vi "GUI_TEA_HPD.vi"() -> ()   [LabVIEW 2013]
uses:
  shared programs/GUI_Template/GUI_master/tcp_new_data_event.ctl
  shared programs/GUI_Template/GUI_master/tcp new data cluster.ctl
  General/shared/Image GUI options.ctl
  Device Driver/FilterWheels/posTypDef.ctl
panel:
  in  "pos.Channel2::6":T1=enum."3" caption="M3_HPD near FilterWheel"
  in  "pos.Channel1::6":T1=enum."3" caption="M3_HPD FilterWheel"
  in  "GUIdevice 6":string="BELLA_filter_wheels"
  in  "Target.X::2":dbl=0.001 caption="X" min=0.0 max=2000.0
  in  "Target.Y::2":dbl=0.001 caption="Y" min=0.0 max=2000.0
  in  "size2":dbl=25.0 caption="Size" min=0.0 max=0.0
  in  "Target.X::5":dbl=0.001 caption="X" min=0.0 max=2000.0
  in  "Target.Y::5":dbl=0.001 caption="Y" min=0.0 max=2000.0
  in  "size5":dbl=25.0 caption="Size" min=0.0 max=0.0
  in  "Image options":T2
  in  "Image options":T2
  in  "GUIdevice 1":string="BELLA_TEA_PowerMeter"
  in  "Reading::1":dbl=0.5 caption="Power (W)" min=0.0 max=50000.0 format="%_4p"
  in  "stop":bool
  out "power":dbl=9999.0 caption="Power (W)" min=0.0 max=300000000.0 format="%_4p"
  in  "Clear":bool
  out "XY Graph":cluster{dbl[], dbl[]}(graph)
  in  "trigger::2":bool caption="Blank Button"
  in  "exposure::2":dbl=0.001 caption="Exposure" min=3.8e-05 max=1.0 format="%_4p"
  out "Display2":T3(plugin-control) caption="M3HPD_CCD"
  in  "GUIdevice 2":string="M3HPD_CCD"
  out "image::2":T3(plugin-control) caption="M1 Cam"
  in  "trigger::5":bool caption="Blank Button"
  in  "exposure::5":dbl=0.001 caption="Exposure" min=3.8e-05 max=1.0 format="%_4p"
  out "Display5":T3(plugin-control) caption="M3HPD_CCD_Near"
  in  "GUIdevice 5":string="M3HPD_CCD_Near"
  out "image::5":T3(plugin-control) caption="M1 Cam"
  out "error IO 2":errorcluster
  out "tcp data event":T4
  # "BELLA TEA HPD MAP"
  # "TEA Power Meter"
  # "Target"
  # "Target"
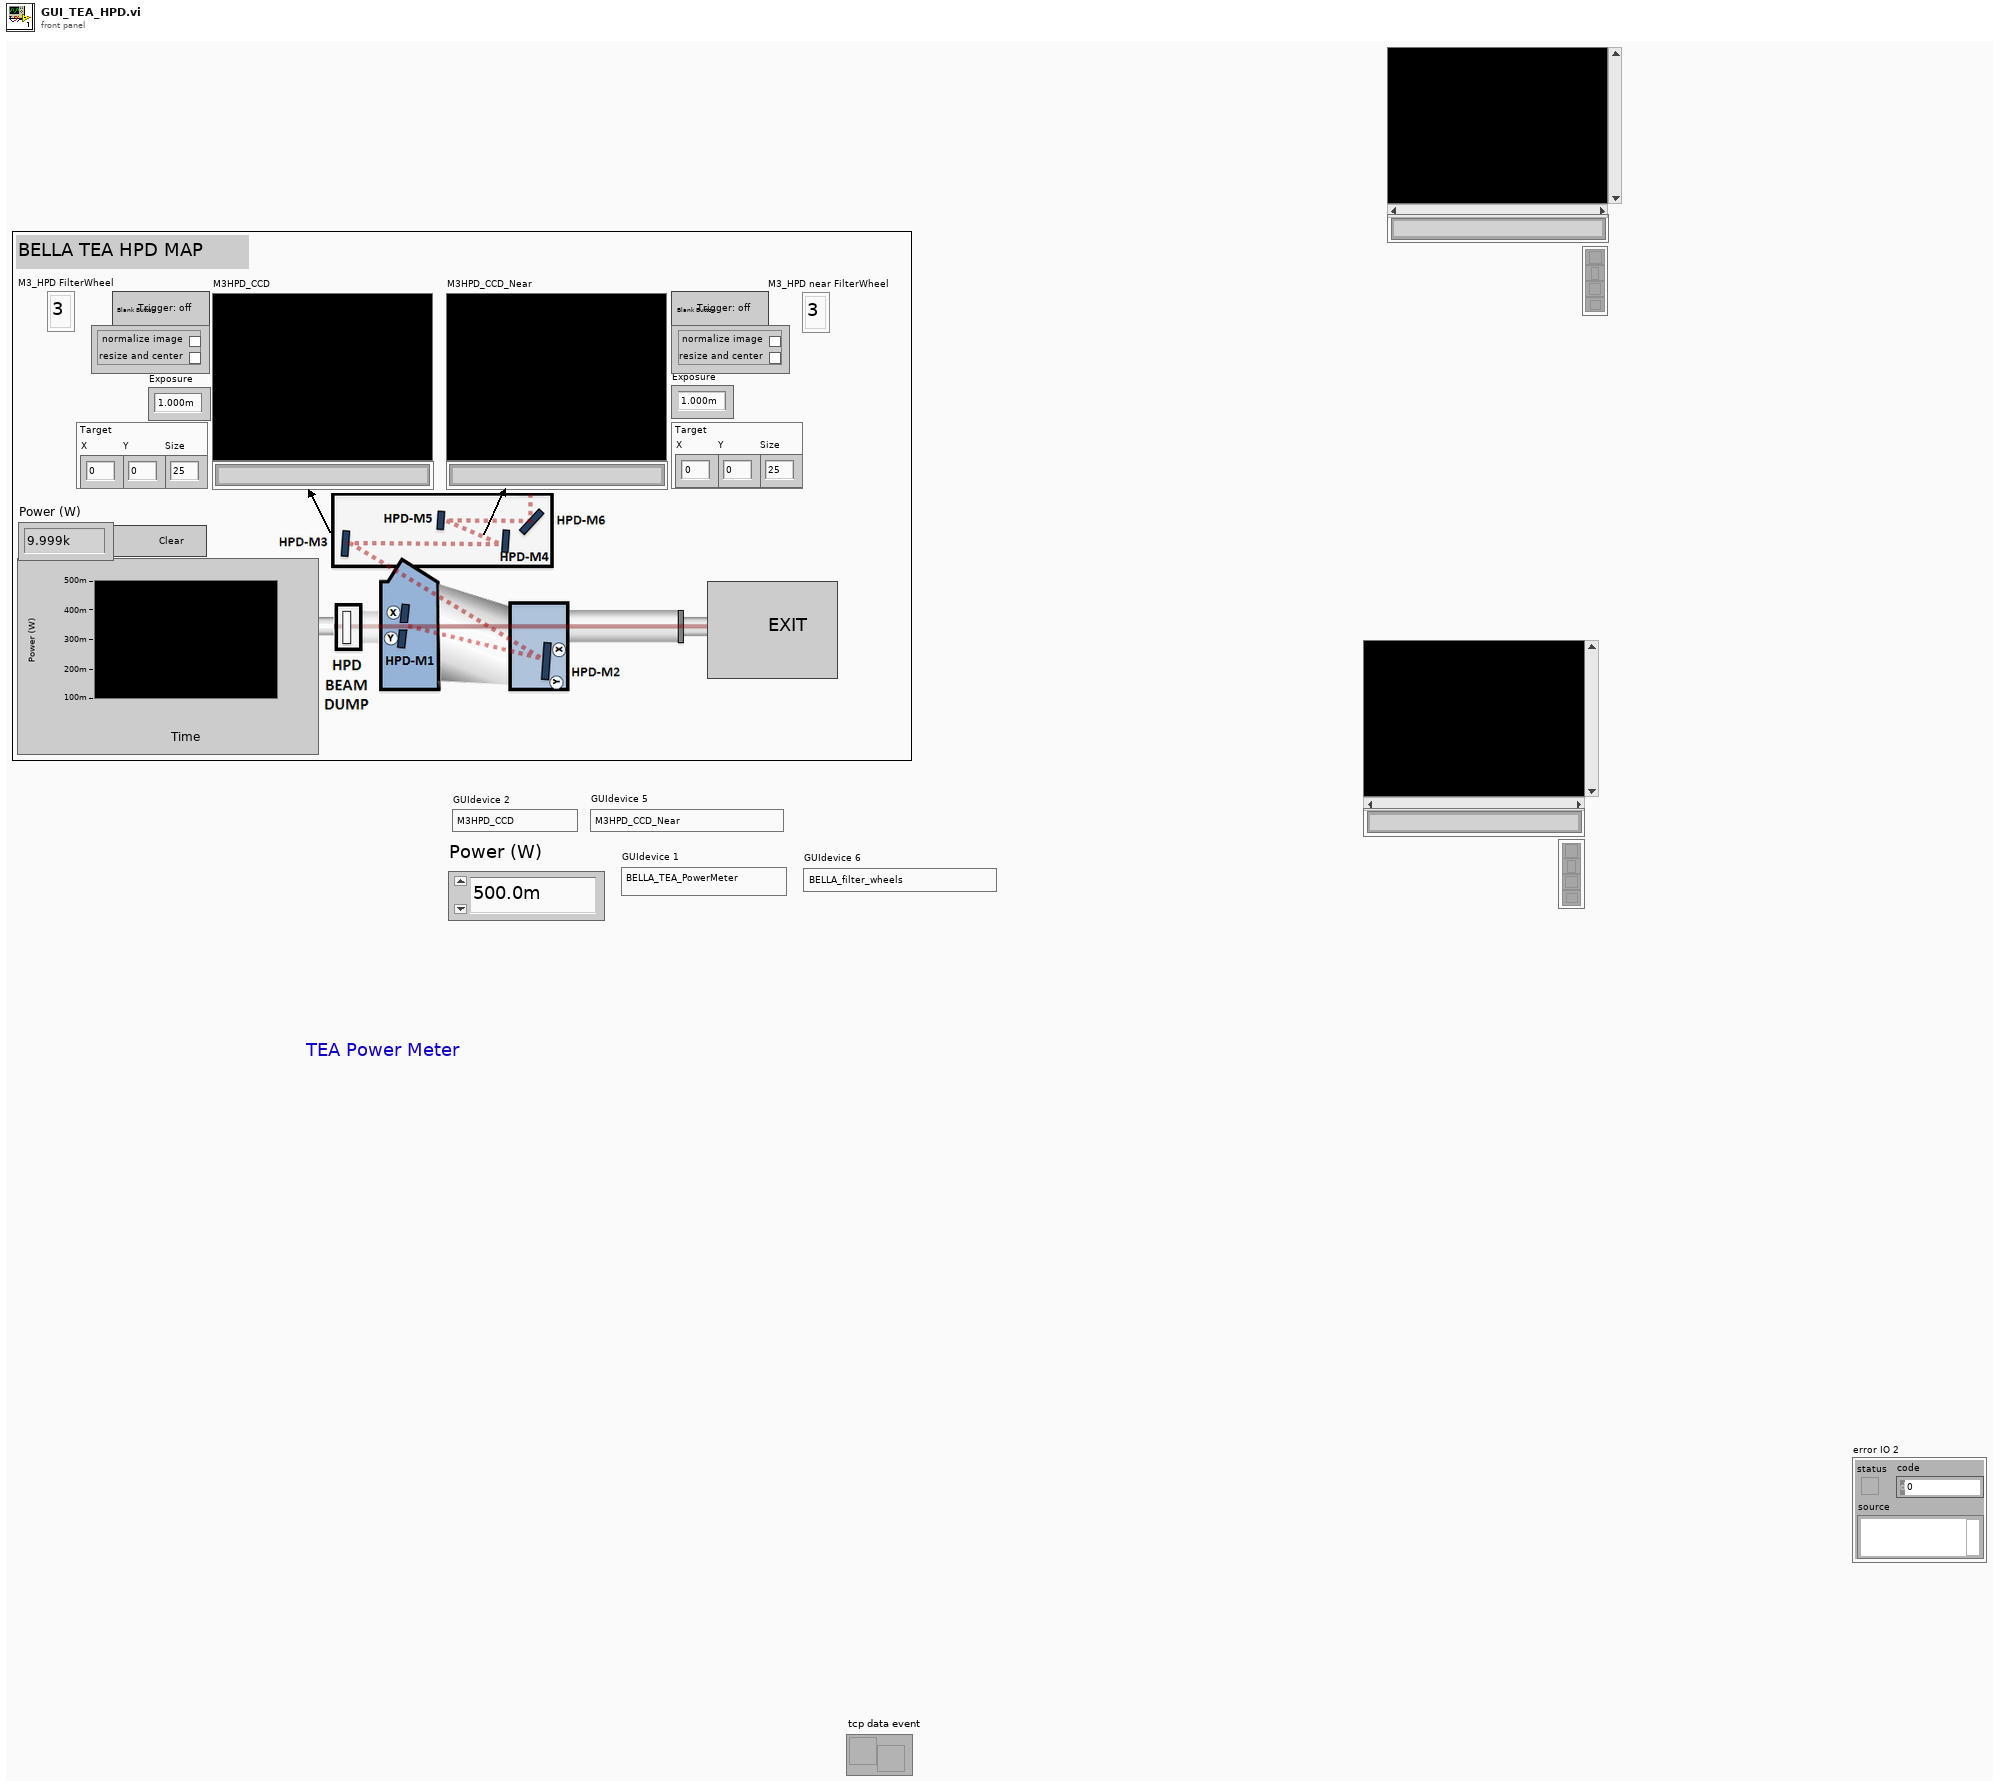
[diagram p1: front panel]
types:
  T1 = typedef "posTypDef.ctl" = enum16{"1", "2", "3", "4", "5", "6"}
  T2 = typedef "Image GUI options.ctl" = cluster{"normalize image":bool, "resize and center":bool}
  T3 = typedef "IMAQ Image.ctl" = refnum<image>
  T4 = typedef "tcp_new_data_event.ctl" = refnum<user-event>
  T5 = typedef "Image Type" = u32
  T6 = typedef "tcp new data cluster.ctl" = cluster{"EventEnum":enum16{"new data", "connection status update"}, "Device name":string}
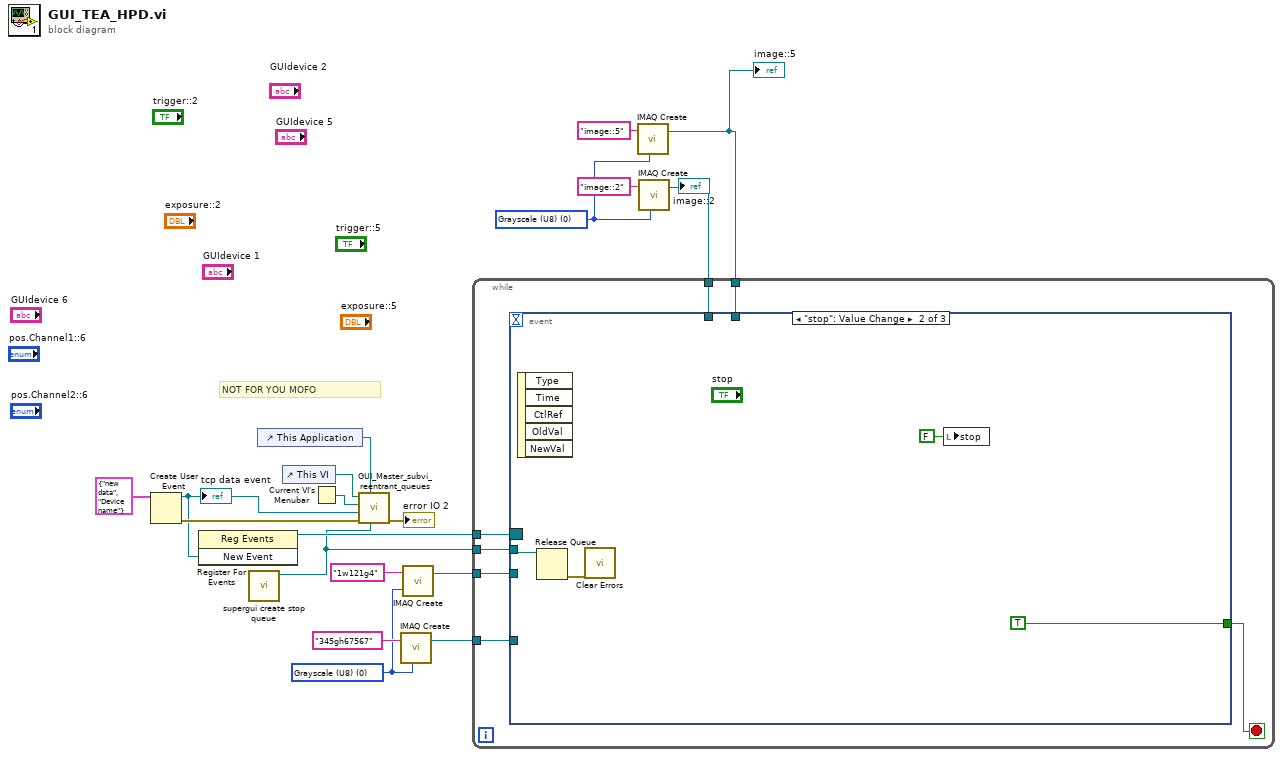
[diagram p0: block diagram]
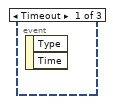
[diagram p2: hidden frame]
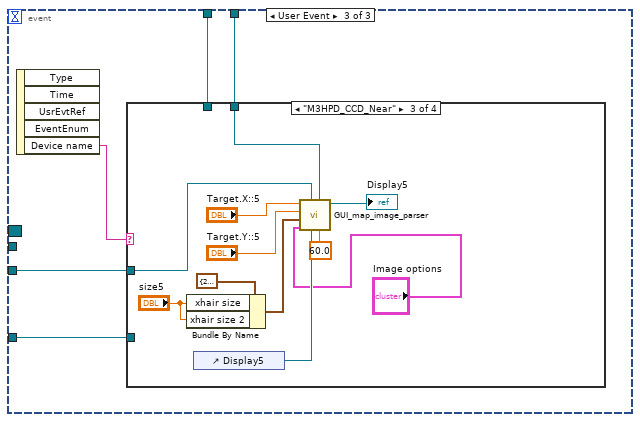
[diagram p3: hidden frame]
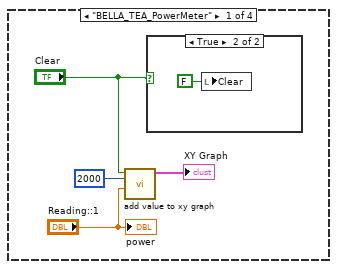
[diagram p4: hidden frame]
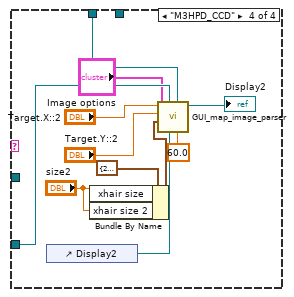
[diagram p7: hidden frame]
diagram:
  w2 = T5 0 items=["Grayscale (U8)", "Grayscale (I16)", "Grayscale (SGL)", "Complex (CSG)", "RGB (U32)", "HSL (U32)", "RGB (U64)", "Grayscale (U16)"] ("Image Type")
  w8 = T5 0 items=["Grayscale (U8)", "Grayscale (I16)", "Grayscale (SGL)", "Complex (CSG)", "RGB (U32)", "HSL (U32)", "RGB (U64)", "Grayscale (U16)"] ("Image Type")
  # "NOT FOR YOU MOFO"
  n1 = Create User Event(user event datatype=T6 {"EventEnum"=enum."new data", "Device name"="Device name"} ("New Event")) -> (user event=w14:refnum<user-event>, error out=w15:errorcluster)  [unwired: 1 in]
  "tcp data event" <- w14
  n2 = register-events(w14) -> (reference out=w12:refnum<event-registration>)  [unwired: 2 in, 1 out]
  n3 = call "supergui create stop queue.vi"() -> ("STOP Queue out"=w1:refnum<queue>)  [unwired: 11 in]
  n4 = control-ref of="This Application"() -> (w13:refnum<vi>)
  n5 = control-ref of="This VI"() -> (w18:refnum<vi>)
  n6 = Current VI's Menubar() -> (w17:refnum<k9>)
  n7 = call "GUI_Master_subvi_reentrant_queues.vi"("STOP Queue in"=w1, "This Application"=w13, "error in (no error)"=w15, "tcp data event"=w14, "Caller menu reference"=w17, "Caller VI ref"=w18) -> ("error out"=→"error IO 2":errorcluster)  [unwired: 5 in]
  n8 = call "IMAQ Create"("Image Name"="345gh67567", "Image Type"=w8) -> ("New Image"=w10:T3)  [unwired: 3 in, 1 out]
  n9 = call "IMAQ Create"("Image Name"="1w121g4", "Image Type"=w8) -> ("New Image"=w7:T3)  [unwired: 3 in, 1 out]
  n10 = call "IMAQ Create"("Image Name"="image::5", "Image Type"=w2) -> ("New Image"=w5:T3)  [unwired: 3 in, 1 out]
  "image::5" <- w5
  n11 = call "IMAQ Create"("Image Name"="image::2", "Image Type"=w2) -> ("New Image"=w3:T3)  [unwired: 3 in, 1 out]
  "image::2" <- w3
  n12 = while {
    tunnel: w12 -> [w25]
    tunnel: w10 -> [w24]
    tunnel: w7 -> [w23]
    tunnel: w5 -> [w22]
    tunnel: w3 -> [w21]
    tunnel: w1 -> [w20]
    stop <- w26 stop-if-true
    n13 = event shown="[1] \"stop\": Value Change" {
      selector: w25 -> [_ _ _]
      dyn-events: _ -> [_ _ _]
      timeout: _ -> [_ _ _]
      tunnel: [_ TRUE _] -> w26
      tunnel: w24 -> [_ _ w34]
      tunnel: w23 -> [_ _ w33]
      tunnel: w22 -> [_ _ w32]
      tunnel: w21 -> [_ _ w31]
      tunnel: w20 -> [_ w28 _]
      event Timeout {
        n14 = event-data() -> ()  [unwired: 1 in, 2 out]
      }
      event "stop": Value Change {
        n15 = event-data() -> ()  [unwired: 1 in, 5 out]
        n16 = Release Queue(queue=w28) -> (error out=w27:errorcluster)  [unwired: 2 in, 2 out]
        n17 = call <vilib>:"Clear Errors.vi"("error in (no error)"=w27) -> ()  [unwired: 6 in, 1 out]
        n18 = local write "stop"(FALSE ("stop")) -> ()
      }
      event User Event {
        n19 = event-data() -> ("Device name"=w35:string)  [unwired: 1 in, 4 out]
        n20 = case shown="\"M3HPD_CCD_Near\"" w35 {
          tunnel: w34 -> [_ _ _ w56]
          tunnel: w33 -> [_ _ w51 _]
          tunnel: w32 -> [_ _ w50 _]
          tunnel: w31 -> [_ _ _ w62]
          frame "BELLA_TEA_PowerMeter" {
            n21 = call "add value to xy graph.vi"("new value"="Reading::1", "max points"=2000 ("y"), "Wire in Stop To Clear Graph on Each Run"="Clear") -> ("XY Graph"=→"XY Graph":cluster{dbl[], dbl[]})  [unwired: 8 in]
            n22 = case shown="True" "Clear" {
              frame False {
              }
              frame True {
                n23 = local write "Clear"(FALSE ("Clear")) -> ()
              }
            }
            "power" <- "Reading::1"
          }
          frame Default {
          }
          frame "M3HPD_CCD_Near" {
            n24 = Bundle By Name(cluster=cluster{"xhair size":dbl, "xhair size 2":dbl} {"xhair size"=20.0, "xhair size 2"=20.0} ("size"), "xhair size"="size5", "xhair size 2"="size5") -> (w42:cluster{"xhair size":dbl, "xhair size 2":dbl})
            n25 = control-ref of="Display5"() -> (w47:refnum<vi>)
            n26 = call "GUI_map_image_parser.vi"("zoom#"=60.0, "Image Src"=w50, "Ctl Refnum"=w47, "Image Dst"=w51, "Image options"="Image options", "size"=w42, "target y"="Target.Y::5", "target x"="Target.X::5") -> ("Img out"=→"Display5":T3)  [unwired: 2 in, 1 out]
          }
          frame "M3HPD_CCD" {
            n27 = control-ref of="Display2"() -> (w59:refnum<vi>)
            n28 = Bundle By Name(cluster=cluster{"xhair size":dbl, "xhair size 2":dbl} {"xhair size"=20.0, "xhair size 2"=20.0} ("size"), "xhair size"="size2", "xhair size 2"="size2") -> (w52:cluster{"xhair size":dbl, "xhair size 2":dbl})
            n29 = call "GUI_map_image_parser.vi"("zoom#"=60.0, "Image Src"=w62, "Ctl Refnum"=w59, "Image Dst"=w56, "Image options"="Image options", "size"=w52, "target y"="Target.Y::2", "target x"="Target.X::2") -> ("Img out"=→"Display2":T3)  [unwired: 2 in, 1 out]
          }
        }
      }
    }
  }
